vi "BarPlotExample1.vi"() -> ()   [LabVIEW 2019, in "HTMLPlot.lvclass"]
uses:
  HTMLPlot.lvclass
  Controls/PlotType.ctl
  Controls/LegendPosition.ctl
  Controls/BarPlotOptions.ctl
  Controls/GenericPlotOptions.ctl
panel:
  in  "Graph 3":refnum<k7>(container)
  out "error out 3":errorcluster
  in  "Graph 2":refnum<k7>(container)
  out "error out 2":errorcluster
  out "error out":errorcluster
  in  "Graph":refnum<k7>(container)
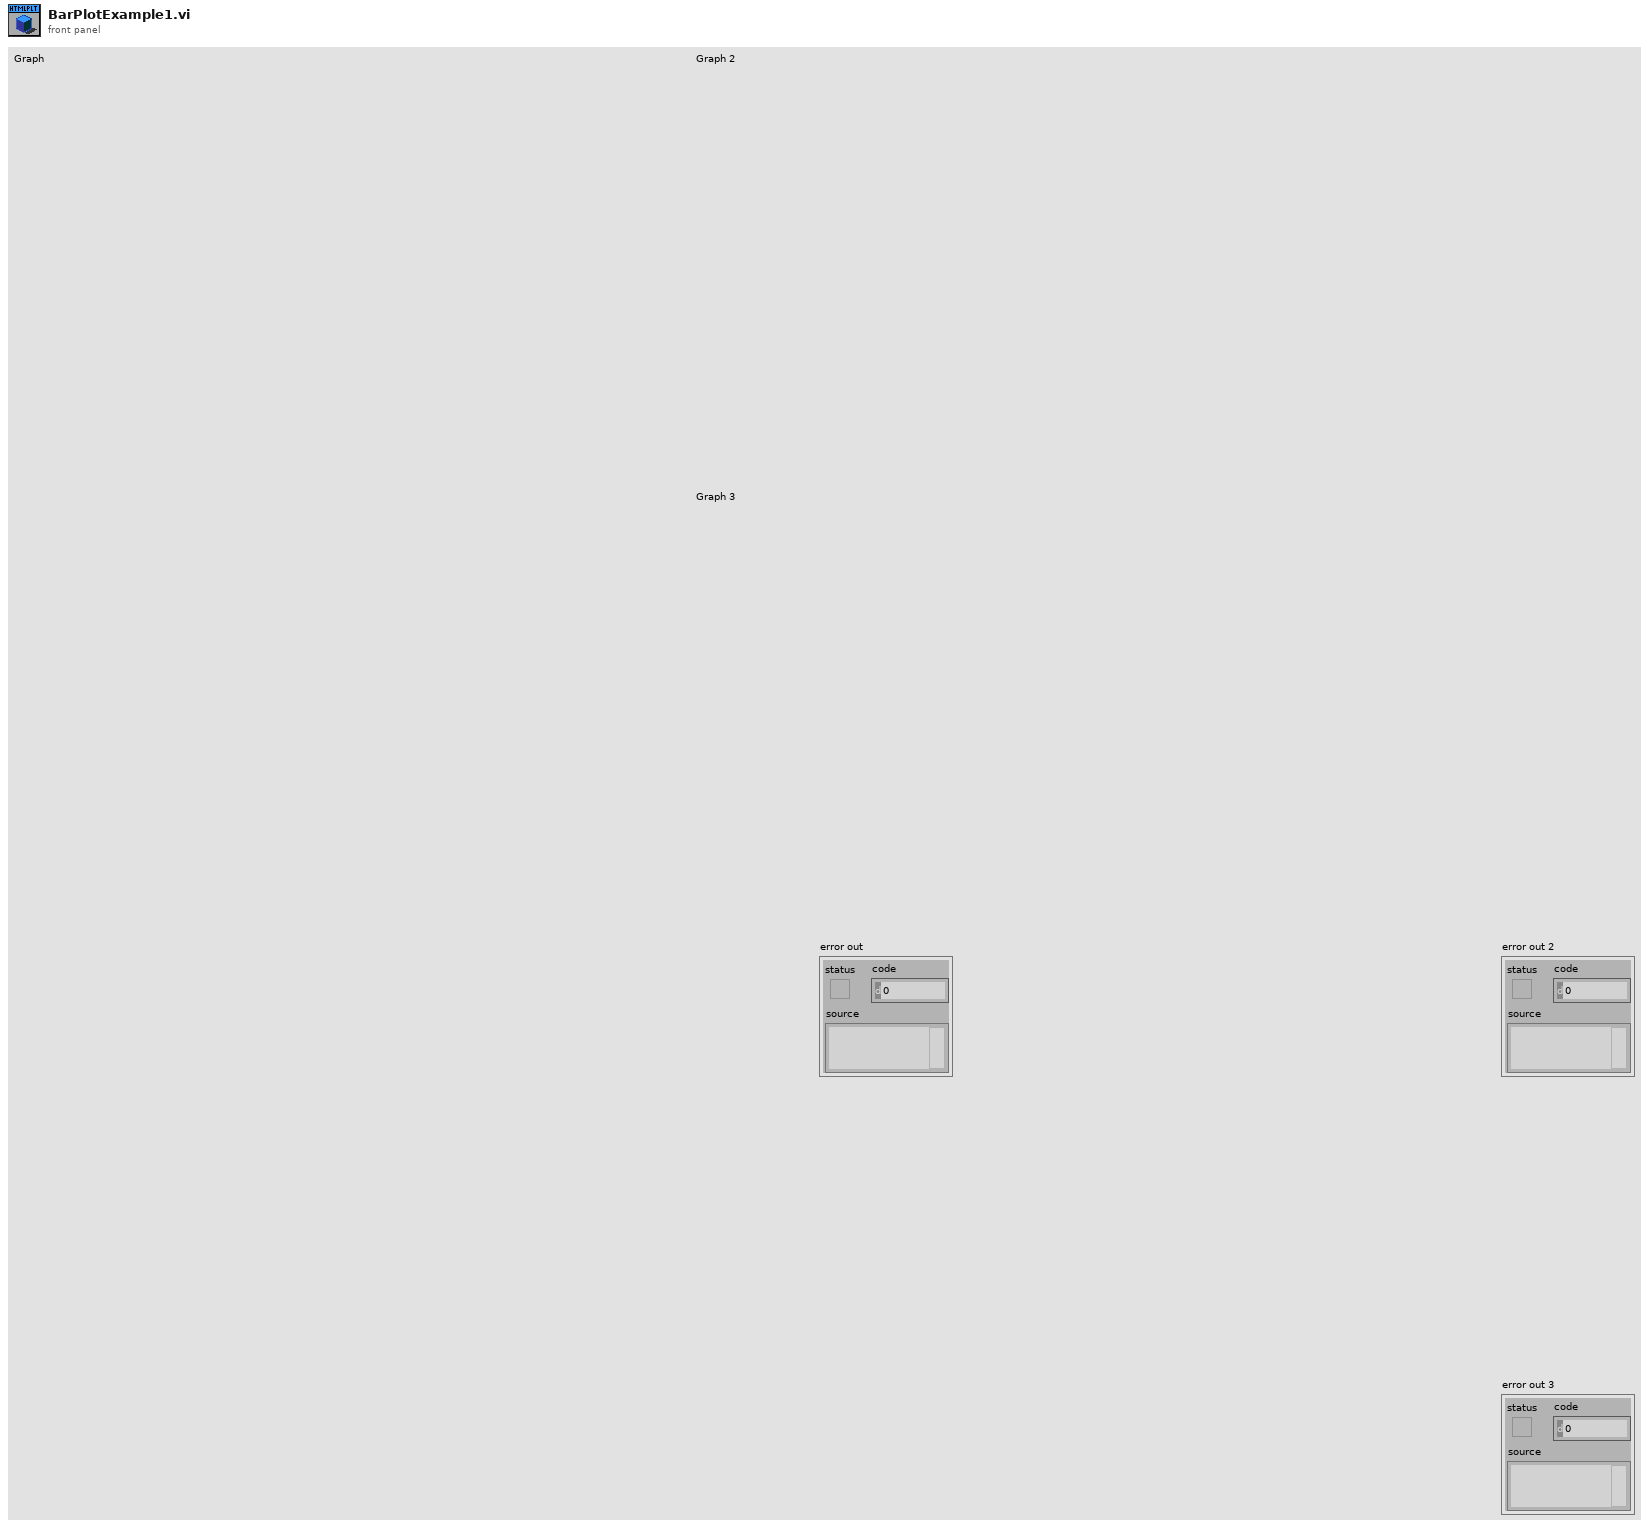
[diagram p1: front panel]
types:
  T1 = typedef "HTMLPlot.lvclass/GenericPlotOptions.ctl" = cluster{"GraphTitle":string, "LegendDisplay":bool, "LegendPosition":T2}
  T2 = typedef "HTMLPlot.lvclass/LegendPosition.ctl" = enum16{"top", "right", "left", "bottom"}
  T3 = typedef "HTMLPlot.lvclass/BarPlotOptions.ctl" = cluster{"xLabel":string, "yLabel":string, "DisplayXLabel":bool, "DisplayYLabel":bool, "Stacked":bool}
  T4 = typedef "HTMLPlot.lvclass/PlotType.ctl" = enum16{"bar", "line", "pie"}
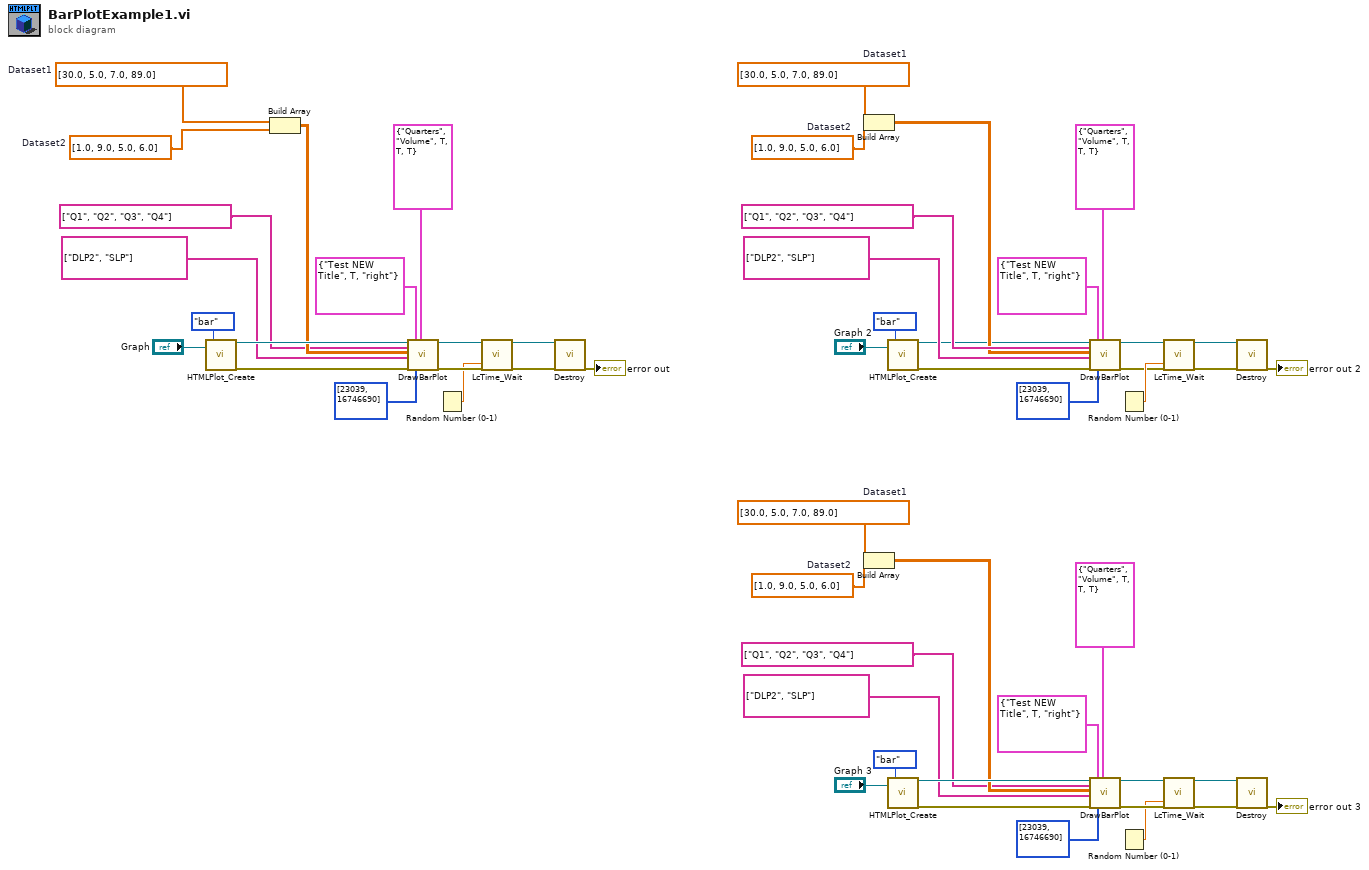
[diagram p0: block diagram]
diagram:
  w14 = dbl[] [1.0, 9.0, 5.0, 6.0]  # Dataset2
  w15 = dbl[] [30.0, 5.0, 7.0, 89.0]  # Dataset1
  w21 = dbl[] [1.0, 9.0, 5.0, 6.0]  # Dataset2
  w20 = dbl[] [30.0, 5.0, 7.0, 89.0]  # Dataset1
  w48 = dbl[] [1.0, 9.0, 5.0, 6.0]  # Dataset2
  w49 = dbl[] [30.0, 5.0, 7.0, 89.0]  # Dataset1
  n1 = call "HTMLPlot_Create.vi"("GraphContainer"="Graph", "PlotType"=PlotType."bar" ("GenericProperties.PlotType")) -> ("reference out"=w46:refnum<class "HTMLPlot.lvclass">, "error out"=w45:errorcluster)  [unwired: 16 in]
  n2 = Build Array(w49, w48) -> (w44:dbl[][])
  n3 = call "DrawBarPlot.vi"("reference in"=w46, "XLabels"=string[] ["Q1", "Q2", "Q3", "Q4"], "BarPlot.Dataset"=w44, "BarPlot.DatasetLabels"=string[] ["DLP2", "SLP"] ("DatasetLabels"), "error in (no error)"=w45, "GenericPlotOptions"=T1 {"GraphTitle"="Test NEW Title", "LegendDisplay"=TRUE, "LegendPosition"=enum."right"}, "BarPlot.PlotColours"=u32[] [23039, 16746690] ("PlotColours"), "BarPlotOptions"=T3 {"xLabel"="Quarters", "yLabel"="Volume", "DisplayXLabel"=TRUE, "DisplayYLabel"=TRUE, "Stacked"=TRUE}) -> ("reference out"=w41:refnum<class "HTMLPlot.lvclass">, "error out"=w40:errorcluster)  [unwired: 10 in]
  n4 = Random Number (0-1)() -> (number: 0 to 1=w35:dbl)
  n5 = call "LcTime_Wait.vi"("secToWait"=w35, "error in (no error)"=w40) -> ("error out"=w36:errorcluster)  [unwired: 15 in, 2 out]
  n6 = call-dynamic "Destroy.vi"("reference in"=w41, "error in (no error)"=w36) -> ("error out"=→"error out":errorcluster)  [unwired: 16 in, 1 out]
  n7 = Build Array(w20, w21) -> (w25:dbl[][])
  n8 = Build Array(w15, w14) -> (w10:dbl[][])
  n9 = call "HTMLPlot_Create.vi"("GraphContainer"="Graph 2", "PlotType"=PlotType."bar" ("GenericProperties.PlotType")) -> ("reference out"=w23:refnum<class "HTMLPlot.lvclass">, "error out"=w24:errorcluster)  [unwired: 16 in]
  n10 = call "HTMLPlot_Create.vi"("GraphContainer"="Graph 3", "PlotType"=PlotType."bar" ("GenericProperties.PlotType")) -> ("reference out"=w12:refnum<class "HTMLPlot.lvclass">, "error out"=w11:errorcluster)  [unwired: 16 in]
  n11 = call "DrawBarPlot.vi"("reference in"=w23, "XLabels"=string[] ["Q1", "Q2", "Q3", "Q4"], "BarPlot.Dataset"=w25, "BarPlot.DatasetLabels"=string[] ["DLP2", "SLP"] ("DatasetLabels"), "error in (no error)"=w24, "GenericPlotOptions"=T1 {"GraphTitle"="Test NEW Title", "LegendDisplay"=TRUE, "LegendPosition"=enum."right"}, "BarPlot.PlotColours"=u32[] [23039, 16746690] ("PlotColours"), "BarPlotOptions"=T3 {"xLabel"="Quarters", "yLabel"="Volume", "DisplayXLabel"=TRUE, "DisplayYLabel"=TRUE, "Stacked"=TRUE}) -> ("reference out"=w28:refnum<class "HTMLPlot.lvclass">, "error out"=w29:errorcluster)  [unwired: 10 in]
  n12 = call "DrawBarPlot.vi"("reference in"=w12, "XLabels"=string[] ["Q1", "Q2", "Q3", "Q4"], "BarPlot.Dataset"=w10, "BarPlot.DatasetLabels"=string[] ["DLP2", "SLP"] ("DatasetLabels"), "error in (no error)"=w11, "GenericPlotOptions"=T1 {"GraphTitle"="Test NEW Title", "LegendDisplay"=TRUE, "LegendPosition"=enum."right"}, "BarPlot.PlotColours"=u32[] [23039, 16746690] ("PlotColours"), "BarPlotOptions"=T3 {"xLabel"="Quarters", "yLabel"="Volume", "DisplayXLabel"=TRUE, "DisplayYLabel"=TRUE, "Stacked"=TRUE}) -> ("reference out"=w7:refnum<class "HTMLPlot.lvclass">, "error out"=w6:errorcluster)  [unwired: 10 in]
  n13 = Random Number (0-1)() -> (number: 0 to 1=w34:dbl)
  n14 = Random Number (0-1)() -> (number: 0 to 1=w1:dbl)
  n15 = call "LcTime_Wait.vi"("secToWait"=w34, "error in (no error)"=w29) -> ("error out"=w33:errorcluster)  [unwired: 15 in, 2 out]
  n16 = call "LcTime_Wait.vi"("secToWait"=w1, "error in (no error)"=w6) -> ("error out"=w2:errorcluster)  [unwired: 15 in, 2 out]
  n17 = call-dynamic "Destroy.vi"("reference in"=w28, "error in (no error)"=w33) -> ("error out"=→"error out 2":errorcluster)  [unwired: 16 in, 1 out]
  n18 = call-dynamic "Destroy.vi"("reference in"=w7, "error in (no error)"=w2) -> ("error out"=→"error out 3":errorcluster)  [unwired: 16 in, 1 out]
